vi "update_position.vi"(8 "error in (no error)":errorcluster, 11 "DL090409StageScaffold in":refnum<class "StageMMS2015ASIfromScientifica.lvclass">) -> (0 "error out":errorcluster, 3 "DL090409StageScaffold out":refnum<class "StageMMS2015ASIfromScientifica.lvclass">)   [LabVIEW 2010, in "StageMMS2015ASIfromScientifica.lvclass"]
uses:
  StageMMS2015ASIfromScientifica.lvclass
  StageDL090409Scaffold/StageDL090409Scaffold/StageDL090409Scaffold.lvclass
  common/classes/ErrorController/ErrorController/class_data.vi
  common/classes/ErrorController/ErrorController/ErrorController.lvclass
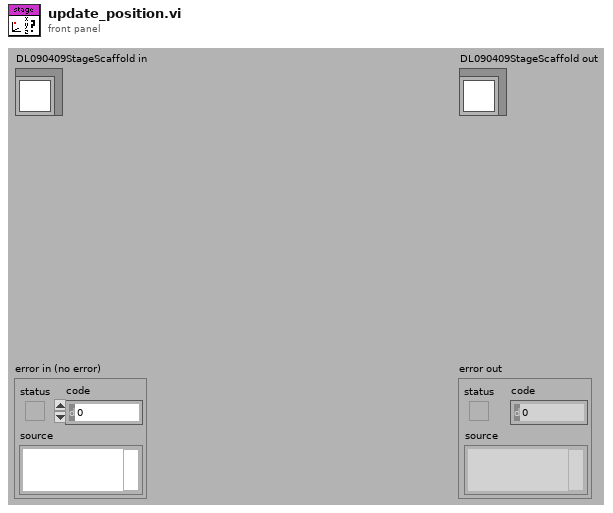
[diagram p1: front panel]
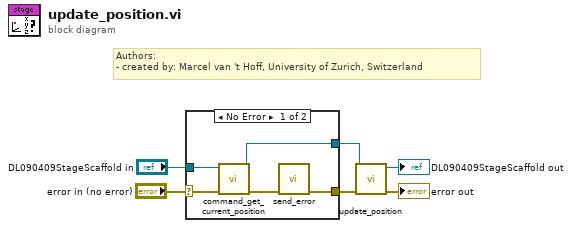
[diagram p0: block diagram]
diagram:
  # "Authors: \n- created by: Marcel van 't Hoff, University of Zurich, Switzerland"
  n1 = case shown="No Error" "error in (no error)" {
    selector: "error in (no error)" -> [w11 w13]
    tunnel: [w9 w13] -> w3
    tunnel: "DL090409StageScaffold in" -> [w8 w12]
    tunnel: [w7 w12] -> w1
    frame No Error {
      n2 = call-dynamic "command_get_current_position.vi"("error in (no error)"=w11, "StageMH110930Scientifica in"=w8) -> ("error out"=w10:errorcluster, "StageMH110930Scientifica out"=w7:refnum<class "StageMMS2015ASIfromScientifica.lvclass">)  [unwired: 7 in, 1 out]
      n3 = call "send_error.vi"("error in (no error)"=w10) -> ("error out"=w9:errorcluster)  [unwired: 10 in]
    }
    frame Error {
    }
  }
  n4 = call-parent "update_position.vi"("error in (no error)"=w3, "DL090409StageScaffold in"=w1) -> ("error out"=→"error out":errorcluster, "DL090409StageScaffold out"=→"DL090409StageScaffold out":refnum<class "StageMMS2015ASIfromScientifica.lvclass">)  [unwired: 8 in]
